vi "check_head_is_neighbour.vi"(1 "head (square knight is sitting on)":T1, 2 "square to check":T3) -> (0 "T = the HEAD is a neighbour":bool)   [LabVIEW 2020, in "core.lvlib"]
uses:
  core.lvlib
  core_data/chessboard_index.ctl
  core_data/chess_square.ctl
  core_data/neighbour_square.ctl
  core_data/core_data.lvlib
panel:
  # "Development\ncontrols/indicators useful for development and testing, but which are not outputs of the VI"
  # "Input\nInputs to the VI"
  # "Output\nOutputs of the VI"
  # "Description\n\nBlank VI with error handling case. \n\nSummarize the use of this VI in this space."
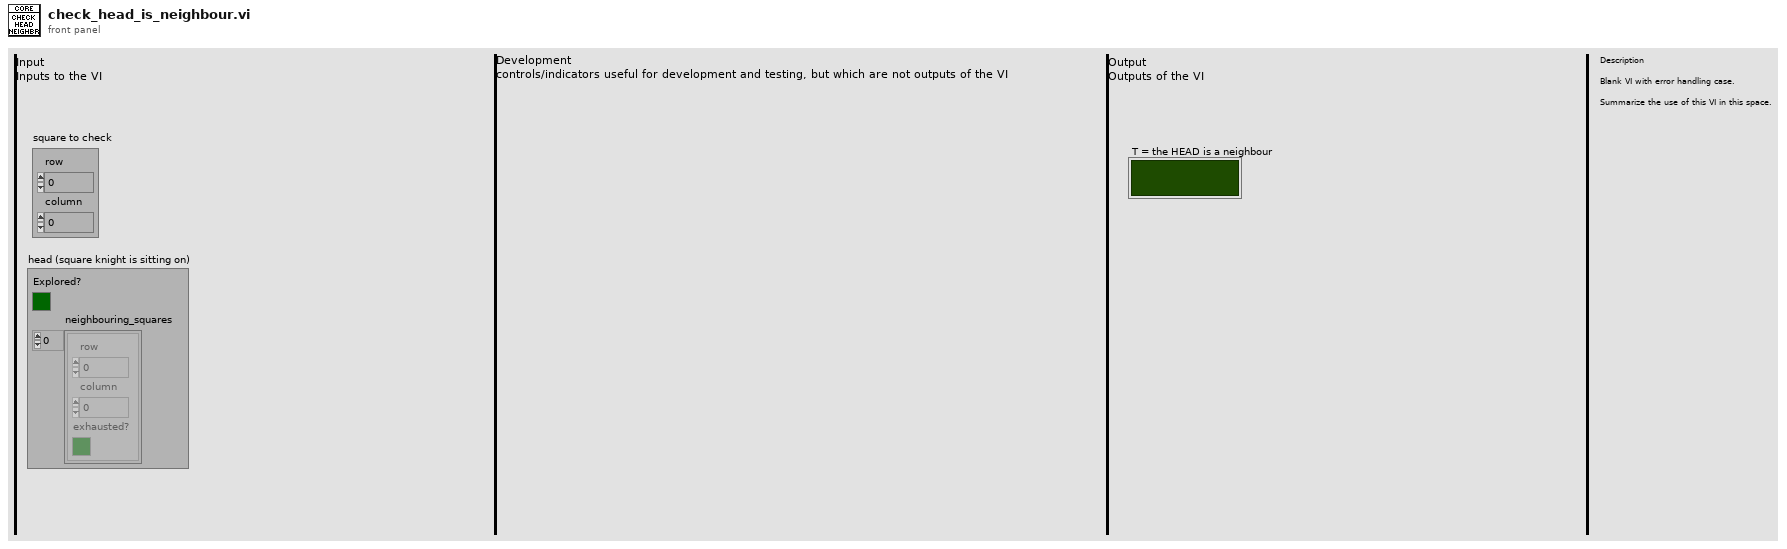
[diagram p1: front panel]
types:
  T1 = typedef "core.lvlib/core_data.lvlib/chess_square.ctl" = cluster{"Explored?":bool, "neighbouring_squares":T2[]}
  T2 = typedef "core.lvlib/core_data.lvlib/neighbour_square.ctl" = cluster{"row":u8, "column":u8, "exhausted?":bool}
  T3 = typedef "core.lvlib/core_data.lvlib/chessboard_index.ctl" = cluster{"row":u8, "column":u8}
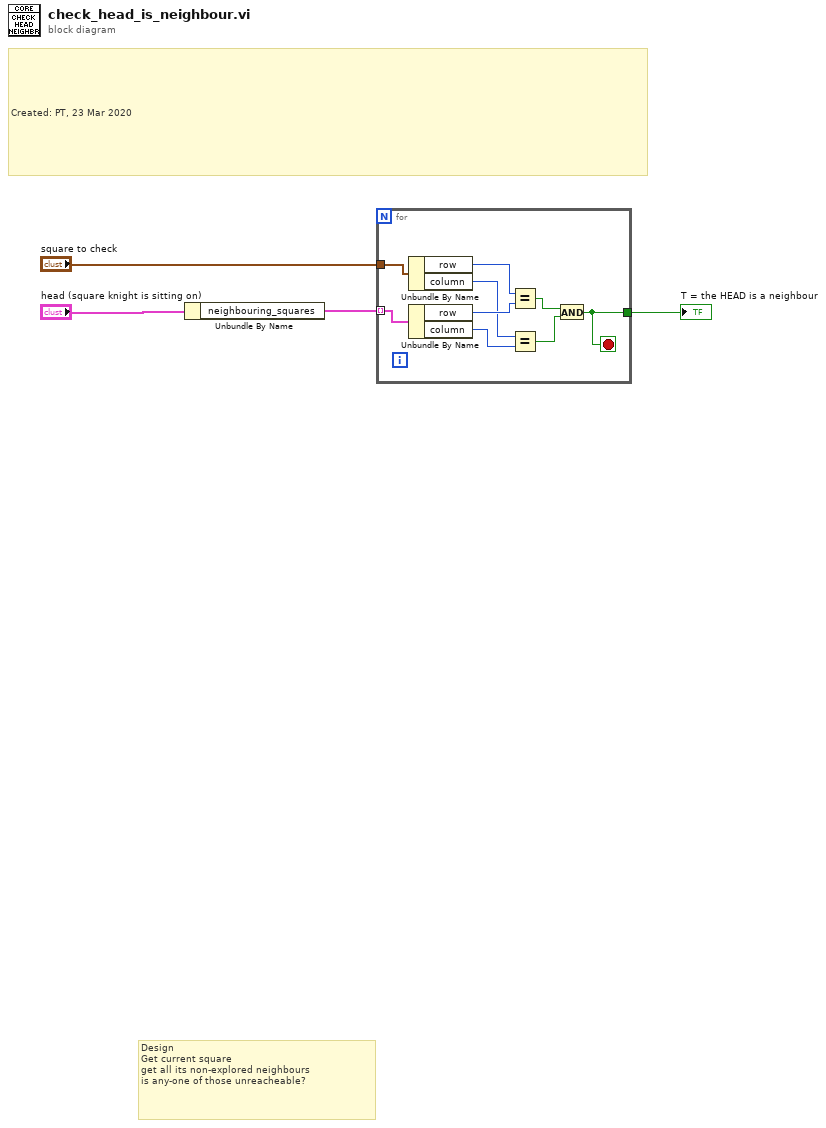
[diagram p0: block diagram]
diagram:
  # "Created: PT, 23 Mar 2020"
  # "Design\nGet current square\nget all its non-explored neighbours\nis any-one of those unreacheable?"
  n1 = Unbundle By Name("head (square knight is sitting on)") -> ("neighbouring_squares"=w4:T2[])
  n2 = for {
    tunnel: w4 -> [w13] mode=indexing
    tunnel: "square to check" -> [w12]
    tunnel: [w5] -> w2
    stop <- w5 stop-if-true
    n3 = Unbundle By Name(w12) -> ("row"=w11:u8, "column"=w9:u8)
    n4 = Unbundle By Name(w13) -> ("row"=w10:u8, "column"=w8:u8)
    n5 = Equal?(x=w11, y=w10) -> (x = y?=w7:bool)
    n6 = Equal?(x=w9, y=w8) -> (x = y?=w6:bool)
    n7 = And(x=w7, y=w6) -> (x .and. y?=w5:bool)
  }
  "T = the HEAD is a neighbour" <- w2
